vi "Bug2 Plan.vi"(0 "RVCLibrary_Bug2 in":refnum<class "RVCLibrary_Bug2.lvclass">, 2 "current reference":refnum<data-value>, 3 "new goal reference":refnum<data-value>, 5 "error in (no error)":errorcluster, 7 "map reference out 2":refnum<data-value>, 8 "overhaul (F)":bool, 9 "epsilon":dbl=1.0) -> (11 "path cost":dbl, 13 "map reference out":refnum<data-value>, 14 "RVCLibrary_Bug2 out":refnum<class "RVCLibrary_Bug2.lvclass">, 15 "path references":refnum<data-value>[](array[refnum]), 16 "no valid path exists":bool, 17 "x":i32, 18 "y":i32, 19 "error out":errorcluster)   [LabVIEW 2013, in "RVCLibrary_Bug2.lvclass"]
uses:
  RVCLibrary_Bug2.lvclass
  <vilib>/robotics/Navigation/shared/MapNode/OccupancyGridNode/NI_Robotics_OccupancyGridMapNode.lvclass
  <vilib>/robotics/Navigation/shared/WorldMap/OccupancyGridWorldMap/NI_Robotics_OccupancyGridWorldMap.lvclass
  <vilib>/robotics/Navigation/NI_Robotics_Navigation .lvlib
  <vilib>/robotics/Navigation/Anytime D Star/NI_Robotics_AnytimeDStar.lvclass
  <vilib>/robotics/Navigation/shared/MapNode/AbstractDstarNode/NI_Robotics_AbstractDstarNode.lvclass
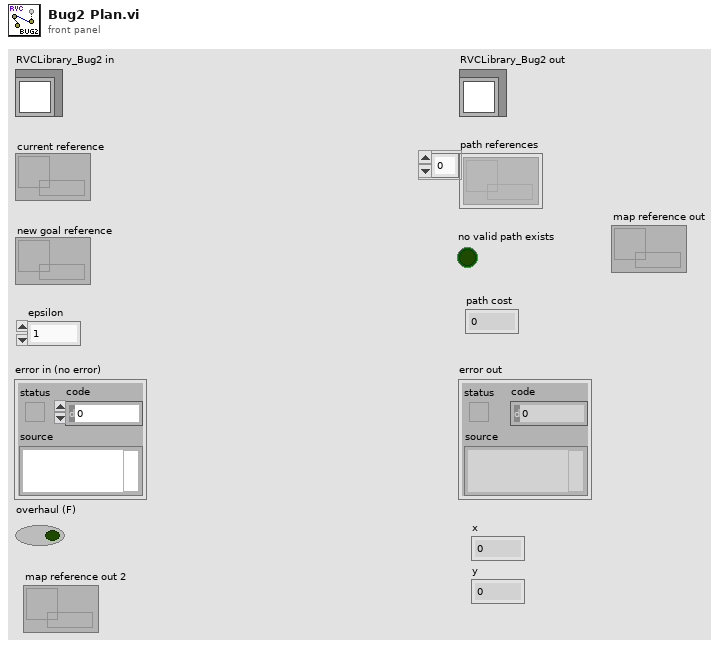
[diagram p1: front panel]
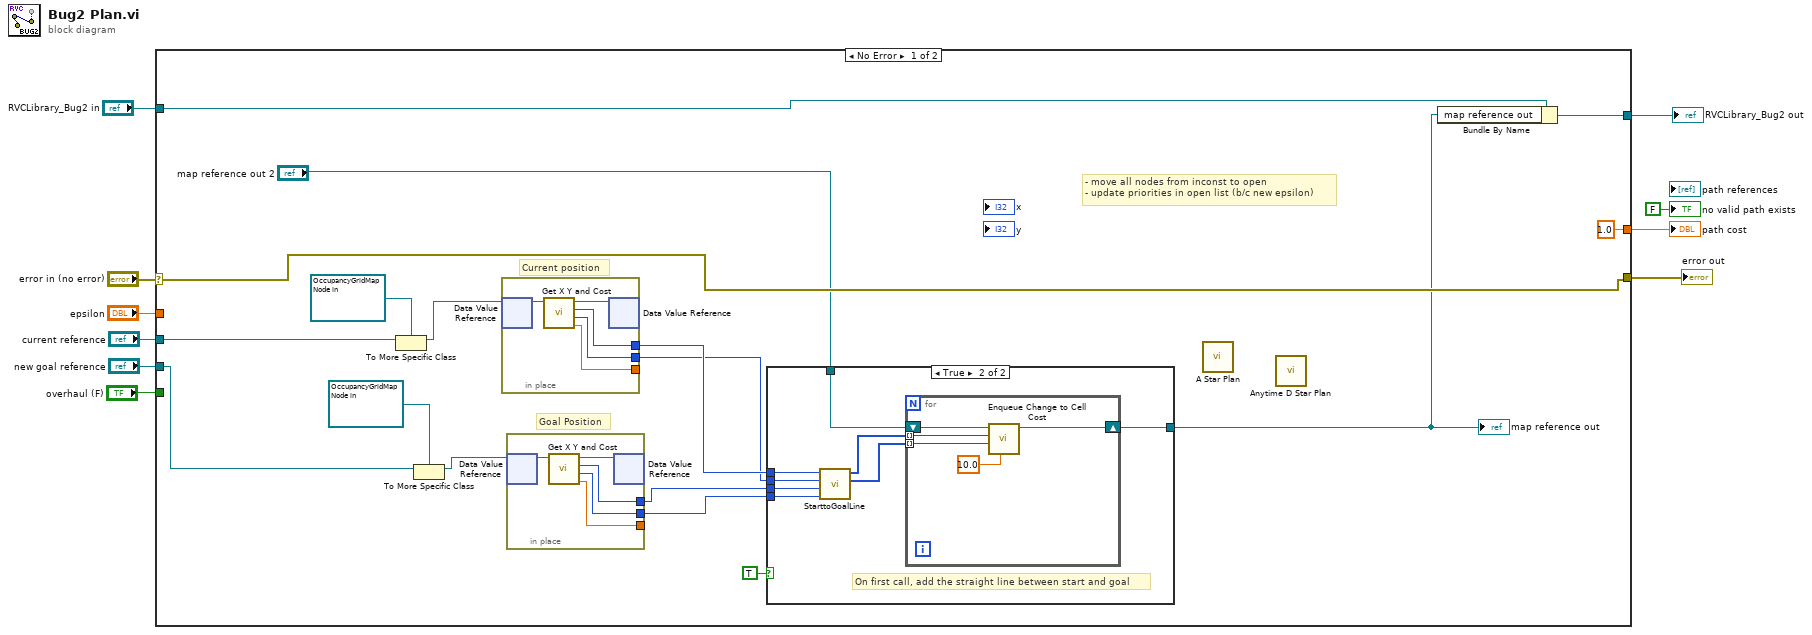
[diagram p0: block diagram]
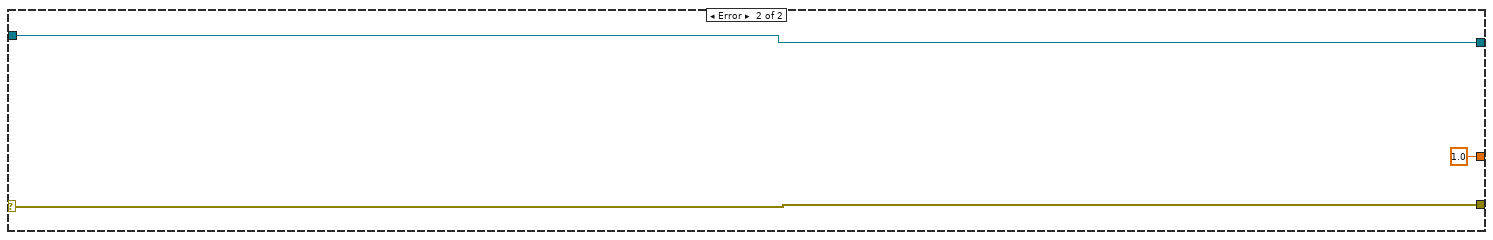
[diagram p3: hidden frame]
diagram:
  n1 = case shown="No Error" "error in (no error)" {
    selector: "error in (no error)" -> [w24 w54]
    tunnel: [w24 w54] -> w9
    tunnel: [w15 w53] -> w8
    tunnel: "RVCLibrary_Bug2 in" -> [w13 w53]
    tunnel: "current reference" -> [w26 _]
    tunnel: "new goal reference" -> [w22 _]
    tunnel: "epsilon" -> [_ _]
    tunnel: "overhaul (F)" -> [_ _]
    tunnel: [1.0 ("path cost") 1.0 ("path cost")] -> w2
    frame No Error {
      # "Goal Position"
      # "Current position"
      # "- move all nodes from inconst to open\n- update priorities in open list (b/c new epsilon)"
      n2 = To More Specific Class(target class=refnum<data-value> refnum ("data value reference"), reference=w26) -> (specific class reference=w25:refnum<data-value>)  [unwired: 1 in, 1 out]
      n3 = To More Specific Class(target class=refnum<data-value> refnum ("data value reference"), reference=w22) -> (specific class reference=w21:refnum<data-value>)  [unwired: 1 in, 1 out]
      n4 = in-place {
        in-place-border: [w50] -> w20
        in-place-border: [w49] -> w19
        in-place-border: [w48] -> _
        n5 = in-place-dvr #1(w25) -> (w51:refnum<class "NI_Robotics_OccupancyGridMapNode.lvclass">)  [unwired: 1 out]
        n6 = call-dynamic "Get X Y and Cost.vi"("OccupancyGridMapNode in"=w51) -> ("Cost"=w48:dbl, "y"=w49:i32, "x"=w50:i32, "OccupancyGridMapNode out"=w47:refnum<class "NI_Robotics_OccupancyGridMapNode.lvclass">)  [unwired: 7 in]
        n7 = in-place-dvr #1(w47) -> ()  [unwired: 2 out]
      }
      n8 = in-place {
        in-place-border: [w45] -> w18
        in-place-border: [w44] -> w17
        in-place-border: [w43] -> _
        n9 = in-place-dvr #2(w21) -> (w46:refnum<class "NI_Robotics_OccupancyGridMapNode.lvclass">)  [unwired: 1 out]
        n10 = call-dynamic "Get X Y and Cost.vi"("OccupancyGridMapNode in"=w46) -> ("Cost"=w43:dbl, "y"=w44:i32, "x"=w45:i32, "OccupancyGridMapNode out"=w42:refnum<class "NI_Robotics_OccupancyGridMapNode.lvclass">)  [unwired: 7 in]
        n11 = in-place-dvr #2(w42) -> ()  [unwired: 2 out]
      }
      n12 = case shown="True" TRUE {
        tunnel: "map reference out 2" -> [w28 w36]
        tunnel: [w28 w33] -> w14
        tunnel: w20 -> [_ w32]
        tunnel: w19 -> [_ w31]
        tunnel: w18 -> [_ w30]
        tunnel: w17 -> [_ w29]
        frame False {
        }
        frame True {
          # "On first call, add the straight line between start and goal"
          n13 = call "StarttoGoalLine.vi"("y1"=w29, "x1"=w30, "y0"=w31, "x0"=w32) -> ("y Line coords"=w34:i32[], "x Line coords"=w35:i32[])  [unwired: 6 in]
          n14 = for {
            shift-right: [w40] -> w33
            shift-left: w36 -> [w41]
            tunnel: w35 -> [w38] mode=indexing
            tunnel: w34 -> [w39] mode=indexing
            n15 = call <vilib>:"Enqueue Change to Cell Cost.vi"("cost"=10.0, "y"=w39, "x"=w38, "map reference in"=w41) -> ("map reference out"=w40:refnum<data-value>)  [unwired: 6 in, 1 out]
          }
        }
      }
      "map reference out" <- w14
      n16 = call <vilib>:"A Star Plan.vi"() -> ()  [unwired: 7 in, 5 out]
      n17 = call <vilib>:"Anytime D Star Plan.vi"() -> ()  [unwired: 7 in, 5 out]
      n18 = Bundle By Name(cluster=w13, "map reference out"=w14) -> (w15:refnum<class "RVCLibrary_Bug2.lvclass">)
    }
    frame Error {
    }
  }
  "error out" <- w9
  "RVCLibrary_Bug2 out" <- w8
  "path cost" <- w2
  "no valid path exists" <- FALSE ("no valid path exists")
